vi "I2C Master(Almost Ready).vi"(4 "Configuration":u8, 5 "Counter":u16=187, 6 "Control":u8, 7 "Address In":u8, 8 "SCL_IN":bool, 9 "SDA_IN":bool, 10 "Execute?":T1, 11 "Data Out":u8) -> (0 "SCL_OUT":bool, 1 "SDA_OUT":bool, 2 "Status":u8, 3 "Data In":u8)   [LabVIEW 2015]
doc: "This VI handles the I2C protocol to transfer data between the master and the slave using Serial Data Line (<b>SDA</b>) and Serial Clock Line (<b>SCL</b>)."
uses:
  Utilities/Start Boolean.ctl
  I2C States.ctl
  I2C Status Signals.ctl
panel:
  # "This VI handles the I2C protocol to transfer data between the master and the slave using Serial Data Line (SDA) and Serial Clock Line (SCL).\n \nI2C Configuration:\nBit [7:1] : Reserved\nBit 0     : Enable or Disable I2C functionality\n \nI2C Control:                                                      I2C Status:\nBit [7:4] : Reserved                                           Bit [7:6] : Reserved\nBit 3     : Data Acknowledge Enable               Bit 5     : I2C bus is busy \nBit 2     : Generate the STOP condition          Bit 4     : I2C subsystem is in use\nBit 1     : Generate the START condition        Bit 3     : Data Not Acknowledge received\nBit 0     : Transmit or receive a data type       Bit 2     : Address Not Acknowledge received\n                                                                            Bit 1     : Error\n                                                                       Bit 0     : I2C subsystem is busy"
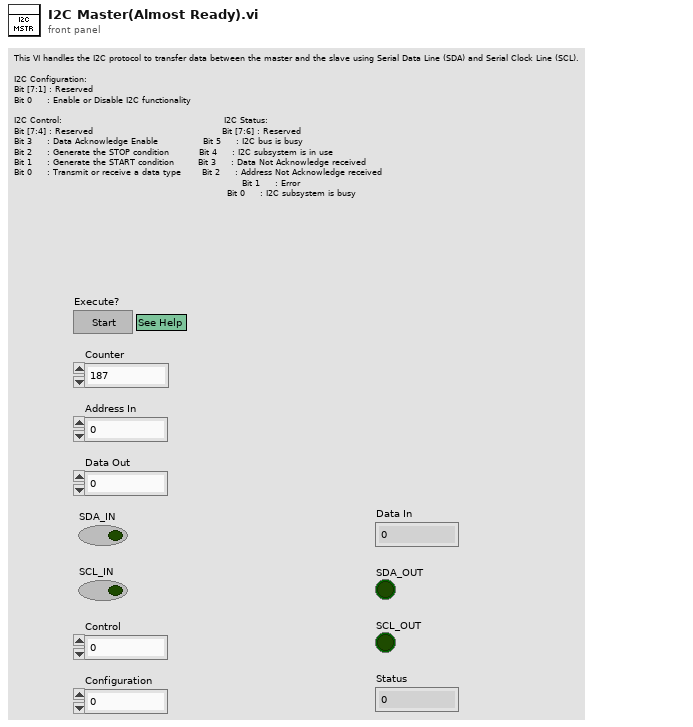
[diagram p1: front panel]
types:
  T1 = typedef "Start Boolean.ctl" = bool
  T2 = typedef "I2C Status Signals.ctl" = cluster{"State":T3, "Timer.Timeout?":bool, "Frame.Complete?":bool, "Data.Address?":bool, "ACK.Address?":bool, "ACK.Stored?":bool}
  T3 = typedef "I2C States.ctl" = fxp<+,5,5>
  T4 = typedef "I2C Configuration.ctl" = cluster{"Enable":bool, "R/S":bool, "Stop":bool, "Start":bool, "Run":bool}
  T5 = typedef "I2C Control Signals.ctl" = cluster{"State+":T3, "Timer.HighPeriod?":bool, "Timer.Load?":bool, "Timer.Increment.":bool, "Frame.LoadSize?":bool, "Frame.Increment":bool, "Data.Address?":bool, "Data.Load":bool, "Data.Setup":bool, "Data.Reset":bool, "Data.Sample":bool, "SDA.Clear":bool, "SDA.Set":bool, "ACK.Sample":bool, "Bus Busy?":bool, "Controller In Use?":bool, "Controller Busy?":bool, "ACK.Store":bool}
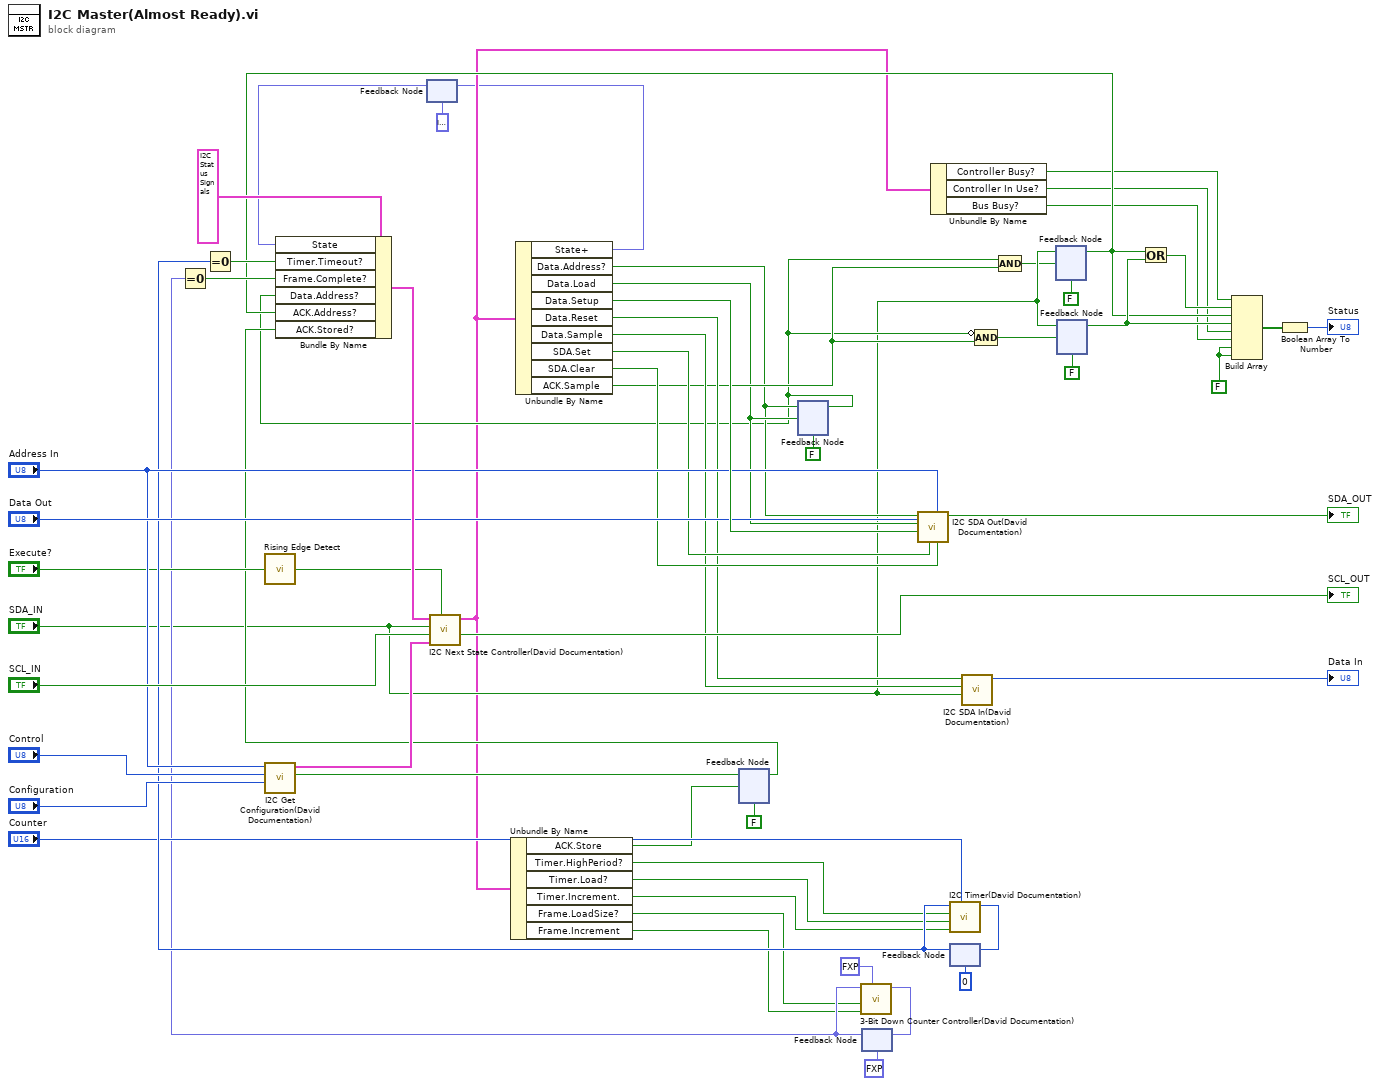
[diagram p0: block diagram]
diagram:
  w41 = FALSE ("element")
  n1 = call "Rising Edge Detect.vi"("Signal"="Execute?") -> ("Trigger?"=w33:bool)
  n2 = call "I2C Get Configuration(David Documentation).vi"("Configuration"="Configuration", "Control"="Control", "Address In"="Address In") -> ("ACK"=w20:bool, "I2C Configuration"=w30:T4)  [unwired: 7 in]
  n3 = feedback #1(T3 0.0 ("State+")) -> (w56:T3)
  n4 = feedback #2(FALSE ("SDA_IN")) -> (w19:bool)
  n5 = feedback #3(FALSE ("SDA_IN")) -> (w15:bool)
  n6 = feedback #4(fxp<+,3,3> 0.0 ("Input")) -> (w27:fxp<+,3,3>)
  n7 = Equal To 0?(x=w27) -> (x = 0?=w54:bool)
  n8 = feedback #5(u16 0 ("Config 2")) -> (w36:u16)
  n9 = Equal To 0?(x=w36) -> (x = 0?=w55:bool)
  n10 = feedback #6(FALSE ("SDA_IN")) -> (w22:bool)
  n11 = Bundle By Name(cluster=T2 {"State"=0.0, "Timer.Timeout?"=FALSE, "Frame.Complete?"=FALSE, "Data.Address?"=FALSE, "ACK.Address?"=FALSE, "ACK.Stored?"=FALSE} ("Status"), "State"=w56, "Timer.Timeout?"=w55, "Frame.Complete?"=w54, "Data.Address?"=w15, "ACK.Address?"=w22, "ACK.Stored?"=w19) -> (w57:T2)
  n12 = call "I2C Next State Controller(David Documentation).vi"("Execute?"=w33, "I2C Configuration"=w30, "SCL_IN"="SCL_IN", "SDA_IN"="SDA_IN", "Status"=w57) -> ("SCL_OUT"=→"SCL_OUT":bool, "Control"=w8:T5)  [unwired: 5 in]
  n13 = Unbundle By Name(w8) -> ("ACK.Store"=w1:bool, "Timer.HighPeriod?"=w7:bool, "Timer.Load?"=w6:bool, "Timer.Increment."=w5:bool, "Frame.LoadSize?"=w4:bool, "Frame.Increment"=w3:bool)
  n14 = Unbundle By Name(w8) -> ("State+"=w2:T3, "Data.Address?"=w16:bool, "Data.Load"=w17:bool, "Data.Setup"=w49:bool, "Data.Reset"=w37:bool, "Data.Sample"=w38:bool, "SDA.Set"=w39:bool, "SDA.Clear"=w40:bool, "ACK.Sample"=w31:bool)
  n15 = feedback-in #1(w2) -> ()
  n16 = feedback-in #2(w20, w1) -> ()
  n17 = feedback-in #3(w16, w17) -> ()
  n18 = call "3-Bit Down Counter Controller(David Documentation).vi"("Input"=fxp<+,3,3> 7.0, "Decrement?"=w3, "Load?"=w4, "Value"=w27) -> ("Value+"=w28:fxp<+,3,3>)  [unwired: 7 in]
  n19 = feedback-in #4(w28) -> ()
  n20 = call "I2C SDA Out(David Documentation).vi"("Clear?"=w40, "Address In"="Address In", "Set?"=w39, "Data In"="Data Out", "Setup?"=w49, "Load?"=w17, "Address?"=w16) -> ("SDA_OUT"=→"SDA_OUT":bool)  [unwired: 4 in]
  n21 = Unbundle By Name(w8) -> ("Controller Busy?"=w11:bool, "Controller In Use?"=w10:bool, "Bus Busy?"=w9:bool)
  n22 = call "I2C Timer(David Documentation).vi"("Counter Value"="Counter", "Decrement?"=w5, "Load?"=w6, "HighPeriod?"=w7, "Value"=w36) -> ("Value+"=w52:u16)  [unwired: 6 in]
  n23 = feedback-in #5(w52) -> ()
  n24 = call "I2C SDA In(David Documentation).vi"("SDA_IN"="SDA_IN", "Sample"=w38, "Reset"=w37) -> ("Data Out"=→"Data In":u8)  [unwired: 8 in]
  n25 = Compound Arithmetic op=AND(invert w15, w31) -> (w13:bool)
  n26 = Compound Arithmetic op=AND(w15, w31) -> (w12:bool)
  n27 = feedback-in #6("SDA_IN", w12) -> ()
  n28 = feedback #7(FALSE ("SDA_IN")) -> (w25:bool)
  n29 = feedback-in #7("SDA_IN", w13) -> ()
  n30 = Or(x=w22, y=w25) -> (x .or. y?=w32:bool)
  n31 = Build Array(w11, w32, w22, w25, w10, w9, w41, w41) -> (w43:bool[])
  n32 = Boolean Array To Number(Boolean array=w43) -> (number=→"Status":u8)
